vi "Initialize Waveforms V2.vi"(0 "SC freq (Hz)":dbl=100000.0, 1 "Amplitude (V)":dbl=1.0 format="%0.2p", 3 "Offset (V)":dbl format="%0.2p", 5 "# lines":i32=256, 7 "line accum":i32=2, 9 "Fast Axis Freq (Hz)":dbl=16208.0 format="%0.2p", 11 "Velocity Limit (V/s)":dbl=-2000.0 format="%0.2p") -> (4 "# lines flyback":i16=40, 6 "total # lines":i32=296, 8 "np":i32=5520, 12 "% active scan":dbl=92.7536231884058, 14 "slow freq (Hz)":dbl=29.36231884057971, 15 "Waveform Values":dbl[](array[numeric]))   [LabVIEW 2014]
panel:
  out "XY Graph":cluster{"t":dbl[], "L":dbl[]}(graph)
  out "dt":dbl=6.169792694965449e-06
  out "T":dbl=0.03405725567620928
  out "t0":dbl=0.032823297137216184
  out "max dh/dt (V/s)":dbl=-1980.1192841578468
  out "constraint":dbl=7537.739130434783
  out "dh":dbl=0.07812500000000001
  out "k":dbl=7463.978793397228
  out "delta t (s)":dbl=0.0024679170779861796
  out "scan slope":dbl=31.656250000000004
  out "t image (s)":dbl=0.0315893385982231
  in  "beta":dbl=0.0001 format="%0.2p"
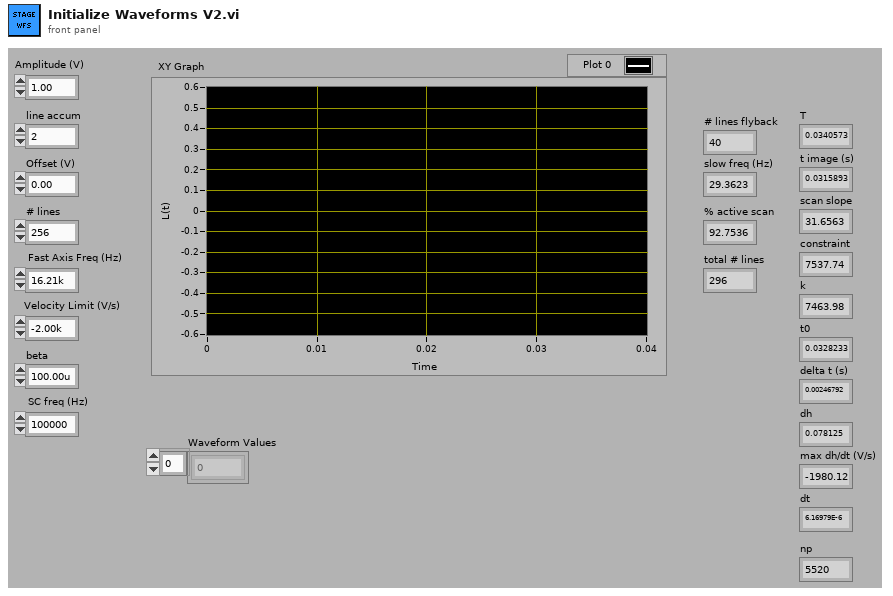
[diagram p1: front panel]
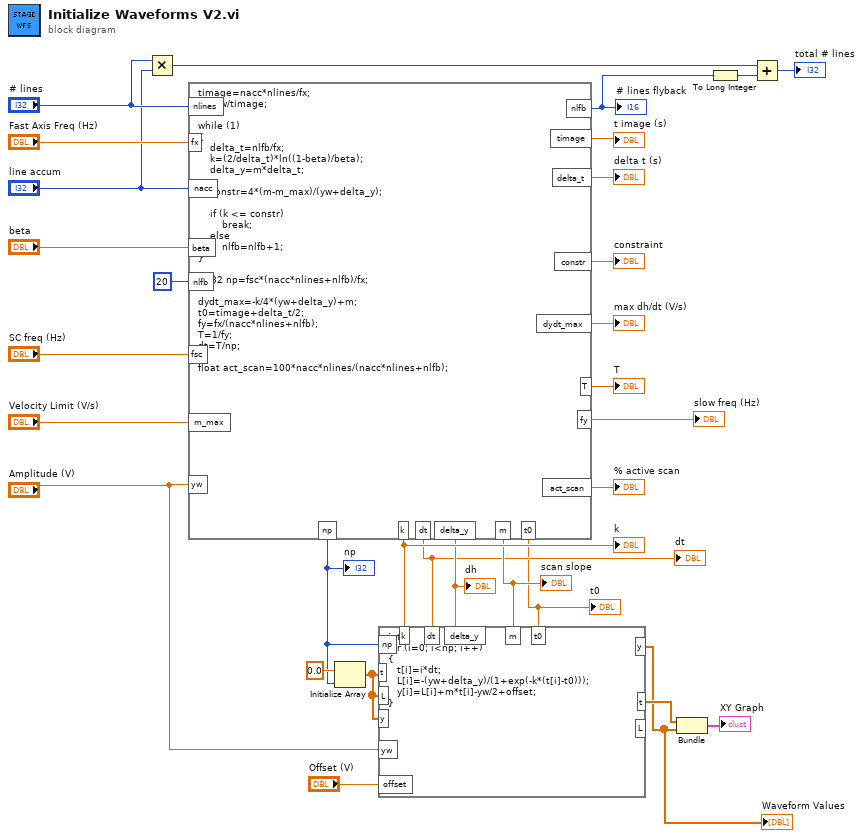
[diagram p0: block diagram]
diagram:
  n1 = Multiply(x="# lines", y="line accum") -> (x*y=w3:i32)
  n2 = formula code="timage=nacc*nlines/fx;\nm=yw/timage; \n\nwhile (1)\n{\n    delta_t=nlfb/fx;\n    k=(2/delta_t)*ln((1-beta)/beta);\n    delta_y=m*delta_t;\n    \n    constr=4*(m-m_max)/(yw+delta_y);\n\n    if (k <= constr)\n        break;\n    else\n        nlfb=nlfb+1;\n}\n\nint32 np=fsc*(nacc*nlines+nlfb)/fx;\n\ndydt_max=-k/4*(yw+delta_y)+m;\nt0=timage+delta_t/2;\nfy=fx/(nacc*nlines+nlfb);\nT=1/fy;\ndt=T/np;\n\nfloat act_scan=100*nacc*nlines/(nacc*nlines+nlfb);"("yw"="Amplitude (V)", "fx"="Fast Axis Freq (Hz)", "nlines"="# lines", "m_max"="Velocity Limit (V/s)", "beta"="beta", "nlfb"=i16 20 ("input variable"), "fsc"="SC freq (Hz)", "nacc"="line accum") -> ("k"=w17:dbl, "delta_t"=→"delta t (s)":dbl, "timage"=→"t image (s)":dbl, "m"=w15:dbl, "delta_y"=w16:dbl, "constr"=→"constraint":dbl, "nlfb"=w9:i16, "dydt_max"=→"max dh/dt (V/s)":dbl, "t0"=w10:dbl, "T"=→"T":dbl, "fy"=→"slow freq (Hz)":dbl, "dt"=w14:dbl, "act_scan"=→"% active scan":dbl, "np"=w18:i32)
  "# lines flyback" <- w9
  "scan slope" <- w15
  "k" <- w17
  "dh" <- w16
  "t0" <- w10
  "dt" <- w14
  "np" <- w18
  n3 = Initialize Array(0.0 ("element"), w18) -> (w20:dbl[])
  n4 = formula code="int i;\nfor (i=0; i<np; i++)\n{\n   t[i]=i*dt;\n   L[i]=-(yw+delta_y)/(1+exp(-k*(t[i]-t0)));\n   y[i]=L[i]+m*t[i]-yw/2+offset;\n}"("np"=w18, "t"=w20, "L"=w20, "y"=w20, "offset"="Offset (V)", "k"=w17, "dt"=w14, "yw"="Amplitude (V)", "delta_y"=w16, "m"=w15, "t0"=w10) -> ("t"=w13:dbl[], "y"=w1:dbl[])  [unwired: 1 out]
  "Waveform Values" <- w1
  n5 = Bundle("t"=w13, "y"=w1) -> (→"XY Graph":cluster{"t":dbl[], "y":dbl[]})  [unwired: 1 out]
  n6 = To Long Integer(number=w9) -> (32bit integer=w6:i32)
  n7 = Add(x=w3, y=w6) -> (x+y=→"total # lines":i32)
